vi "TableCOM.vi"(0 "VISA resource name":refnum<visa-resource-name>) -> (1 "COMSTATUS":bool, 2 "Position 1":string, 3 "Position 2":string)   [LabVIEW 2010]
panel:
  out "Message":string="Le contrôleur des tables \nne répond pas !"
  in  "Réessayer":bool
  in  "OK":bool
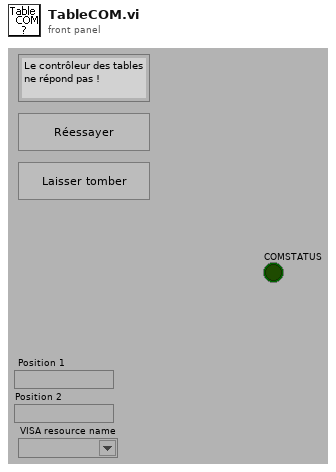
[diagram p1: front panel]
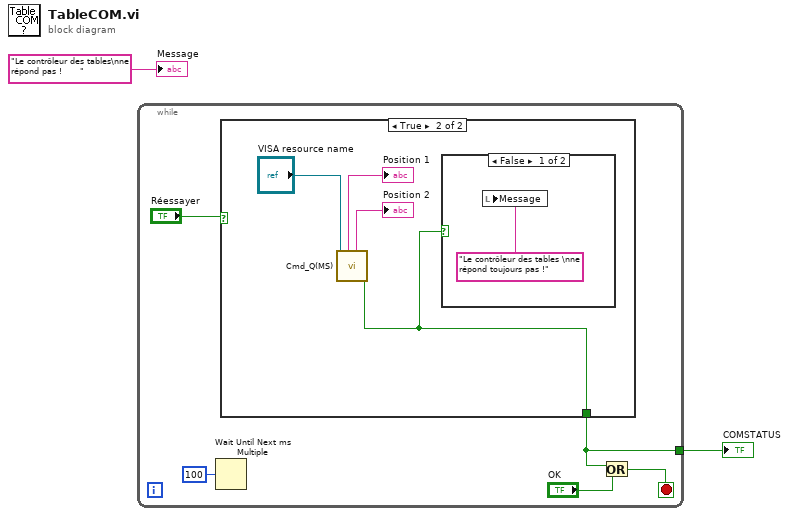
[diagram p0: block diagram]
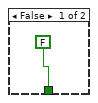
[diagram p2: hidden frame]
diagram:
  n1 = while {
    tunnel: [w3] -> w1
    stop <- w5 stop-if-true
    n2 = Wait Until Next ms Multiple(millisecond multiple=u32 100 ("n millisecondes")) -> ()  [unwired: 1 out]
    n3 = case shown="True" "Réessayer" {
      tunnel: [FALSE w12] -> w3
      frame False {
      }
      frame True {
        n4 = call "Cmd_Q(MS).vi"("VISA resource name IN"="VISA resource name") -> ("OK Done"=w12:bool, "Position 2"=→"Position 2":string, "Position 1"=→"Position 1":string)  [unwired: 3 in, 5 out]
        n5 = case shown="False" w12 {
          frame False {
            n6 = local write "Message"("Le contrôleur des tables \nne répond toujours pas !" ("Message")) -> ()
          }
          frame True {
          }
        }
      }
    }
    n7 = Or(x=w3, y="OK") -> (x .or. y?=w5:bool)
  }
  "COMSTATUS" <- w1
  "Message" <- "Le contrôleur des tables\nne répond pas !      " ("Message")
